vi "Create or Open System Defintion File.vi"(8 "error in (no error)":errorcluster, 10 "File Action":enum16{"Open", "Create"}(ring), 11 "Sysdef File":path) -> (0 "error out":errorcluster, 3 "SysDef Refs":T1)   [LabVIEW 2010]
uses:
  SysDefRefs.ctl
  NationalInstruments.VeriStand.SystemDefinitionAPI
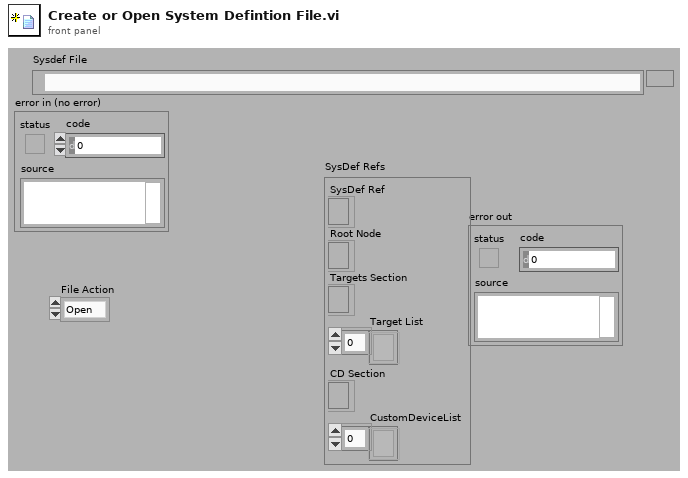
[diagram p1: front panel]
types:
  T1 = typedef "SysDefRefs.ctl" = cluster{"SysDef Ref":refnum<k24>, "Root Node":refnum<k24>, "Targets Section":refnum<k24>, "Target List":refnum<k24>[], "CD Section":refnum<k24>, "CustomDeviceList":refnum<k24>[]}
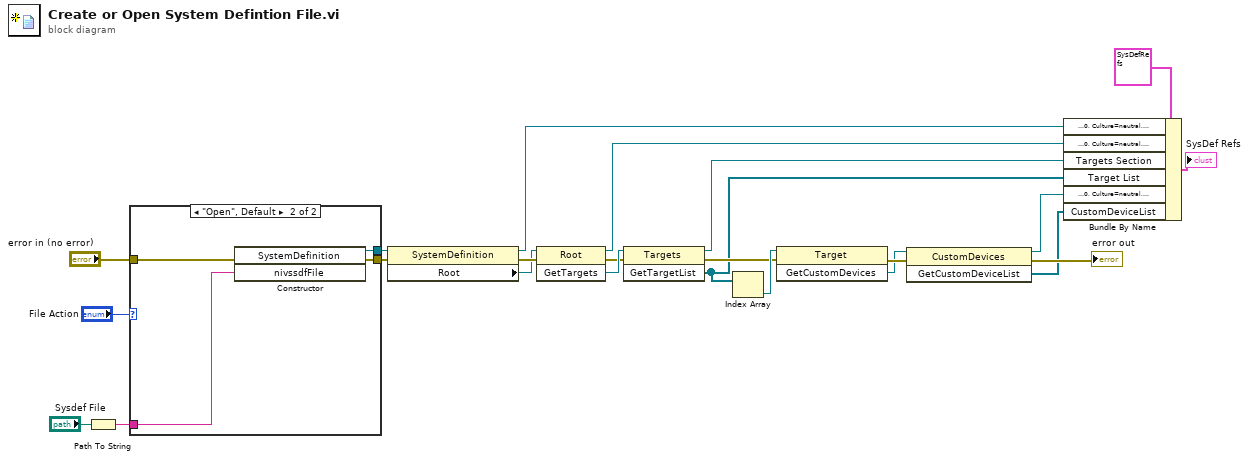
[diagram p0: block diagram]
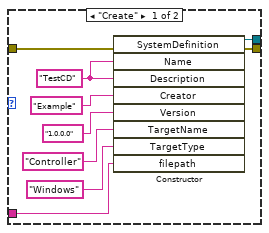
[diagram p2: hidden frame]
diagram:
  n1 = Path To String(path="Sysdef File") -> (string=w18:string)
  n2 = case shown="\"Open\", Default" "File Action" {
    tunnel: [w32 w36] -> w20
    tunnel: [w31 w35] -> w19
    tunnel: w18 -> [w30 w33]
    tunnel: "error in (no error)" -> [w24 w34]
    frame "Create" {
      w25 = "TestCD" ("Name")
      n3 = constructor class="SystemDefinition"(error in=w24, "Name"=w25, "Description"=w25, "Creator"="Example", "Version"="1.0.0.0", "TargetName"="Controller", "TargetType"="Windows", "filepath"=w30) -> (reference out=w31:refnum<k24>, error out=w32:errorcluster)  [unwired: 2 in, 8 out]
    }
    frame "Open", Default {
      n4 = constructor class="SystemDefinition"(error in=w34, "nivssdfFile"=w33) -> (reference out=w35:refnum<k24>, error out=w36:errorcluster)  [unwired: 2 in, 2 out]
    }
  }
  n5 = property class="SystemDefinition"(reference=w19, error in=w20) -> (reference out=w14:refnum<k24>, error out=w22:errorcluster, "Root"=w21:refnum<k24>)
  n6 = invoke class="Root" method="GetTargets"(reference=w21, error in=w22) -> (reference out=w13:refnum<k24>, error out=w16:errorcluster, "GetTargets"=w23:refnum<k24>)  [unwired: 1 in]
  n7 = invoke class="Targets" method="GetTargetList"(reference=w23, error in=w16) -> (reference out=w12:refnum<k24>, error out=w8:errorcluster, "GetTargetList"=w7:refnum<k24>[])  [unwired: 1 in]
  n8 = Index Array(array=w7) -> (element=w9:refnum<k24>)  [unwired: 1 in]
  n9 = invoke class="Target" method="GetCustomDevices"(reference=w9, error in=w8) -> (error out=w5:errorcluster, "GetCustomDevices"=w4:refnum<k24>)  [unwired: 1 in, 1 out]
  n10 = invoke class="CustomDevices" method="GetCustomDeviceList"(reference=w4, error in=w5) -> (reference out=w2:refnum<k24>, error out=→"error out":errorcluster, "GetCustomDeviceList"=w1:refnum<k24>[])  [unwired: 1 in]
  n11 = Bundle By Name(cluster=T1 {"SysDef Ref"=refnum, "Root Node"=refnum, "Targets Section"=refnum, "Target List"=[], "CD Section"=refnum, "CustomDeviceList"=[]} ("SysDef Refs"), "SysDef Ref"=w14, "Root Node"=w13, "Targets Section"=w12, "Target List"=w7, "CD Section"=w2, "CustomDeviceList"=w1) -> (→"SysDef Refs":T1)
